vi "UserMgr-Window.vi"(8 "error in":errorcluster) -> (0 "error out":errorcluster)   [LabVIEW 2017, in "Login-UI.lvlib"]
uses:
  Login-UI.lvlib
  _Typedef/User-Info.ctl
  _Typedef/User-Role.ctl
  2fbc59fa-d6e3-46c3-98fb-aa3f40a50569.vi
  b49018c0-b0cc-4a1e-8c0a-6a6f7b5dc366.vi
  <userlib>/NEVSTOP-Programming-Palette/Configuration/ClusterCfgTable/Parse CfgTable(with DataName).vi
panel:
  in  "Exit":bool
  in  "Edit Button":bool
  in  "Add Button":bool
  in  "Delete Button":bool
  in  "Table":i32(listbox)
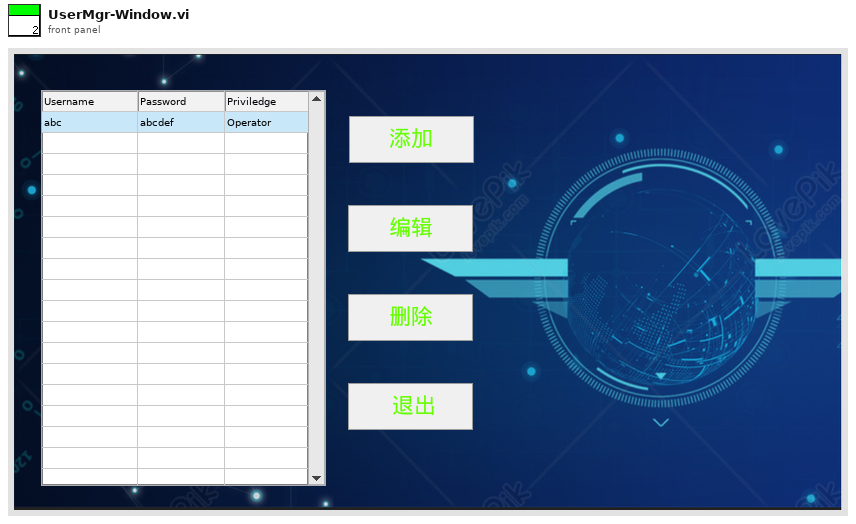
[diagram p1: front panel]
types:
  T1 = typedef "Login-UI.lvlib/User-Info.ctl" = cluster{"UserName":string, "Password":string, "Role":T2}
  T2 = typedef "Login-UI.lvlib/User-Role.ctl" = enum16{"INVALID", "Operator", "Engineer", "Admin"}
  T3 = enum32{"Invalid", "Standard", "Closed", "Hidden", "Minimized", "Maximized"}
  T4 = enum32{"invalid app kind", "Development System", "Run Time System", "Student Edition", "Embedded LabVIEW", "Evaluation", "Custom"}
  T5 = cluster{"Core":cluster{"Current VI Reference":refnum<vi>, "Close Panel on Exit?":bool}, "Your Boolean data":bool, "Your string data":string, "Table Ref":refnum<vi>}
  T6 = cluster{"Current VI Reference":refnum<vi>, "Close Panel on Exit?":bool}
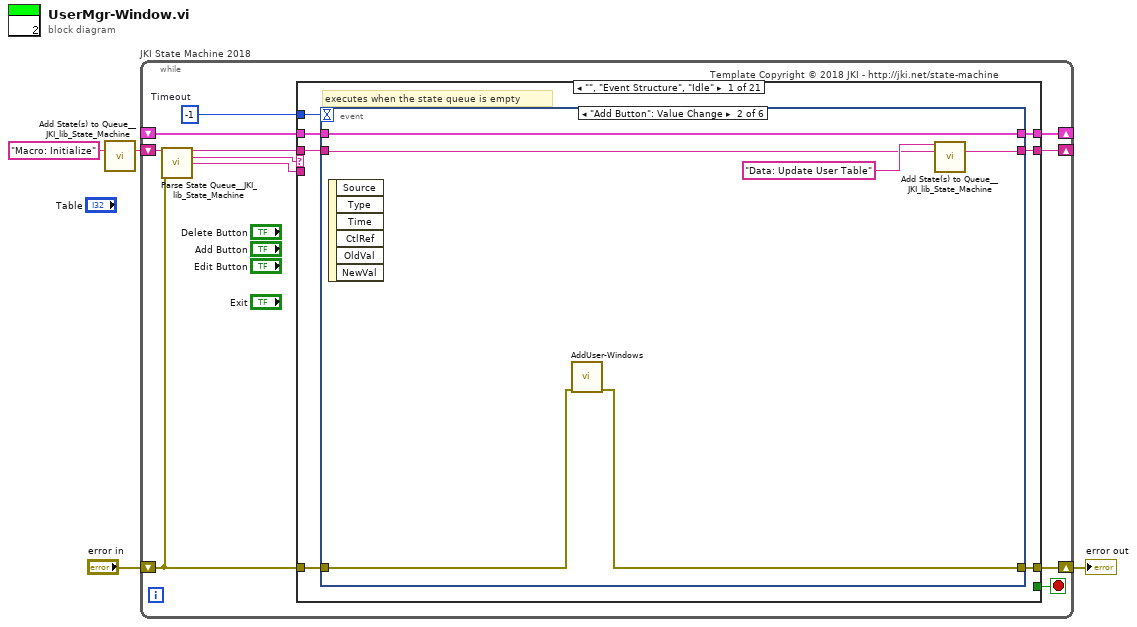
[diagram p0: block diagram]
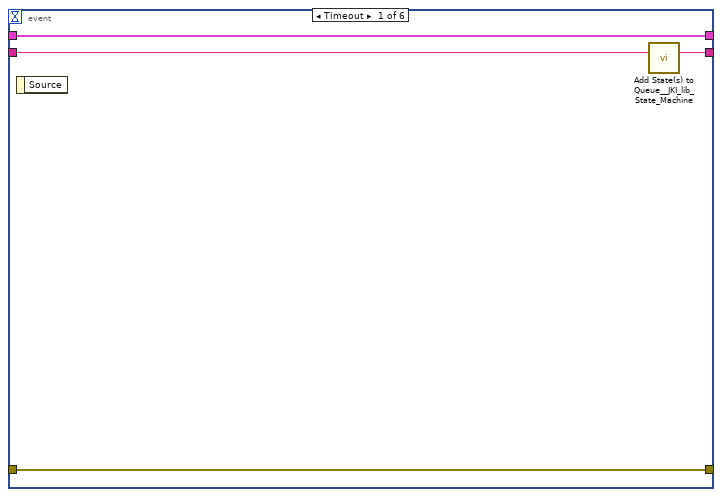
[diagram p2: hidden frame]
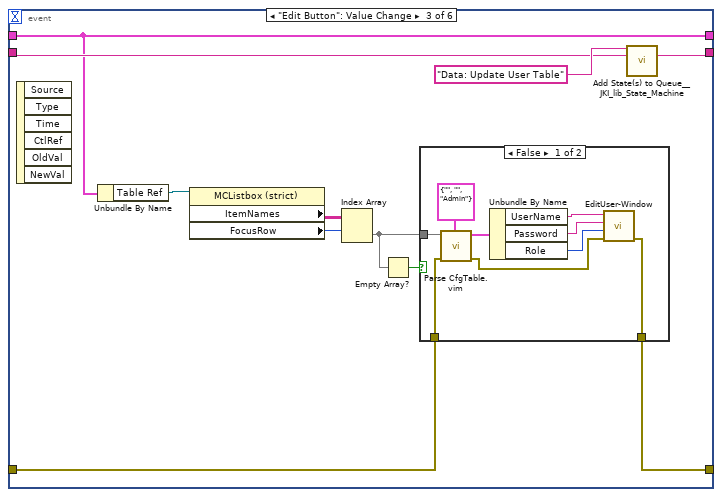
[diagram p3: hidden frame]
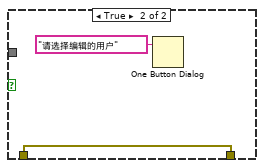
[diagram p4: hidden frame]
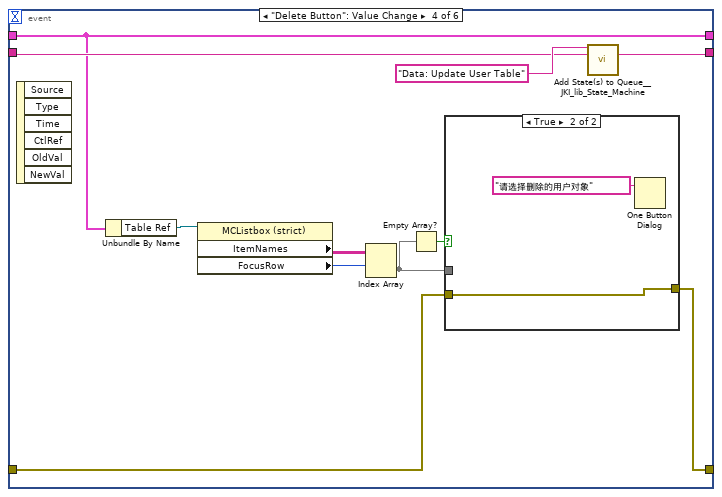
[diagram p5: hidden frame]
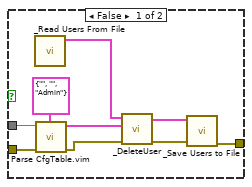
[diagram p6: hidden frame]
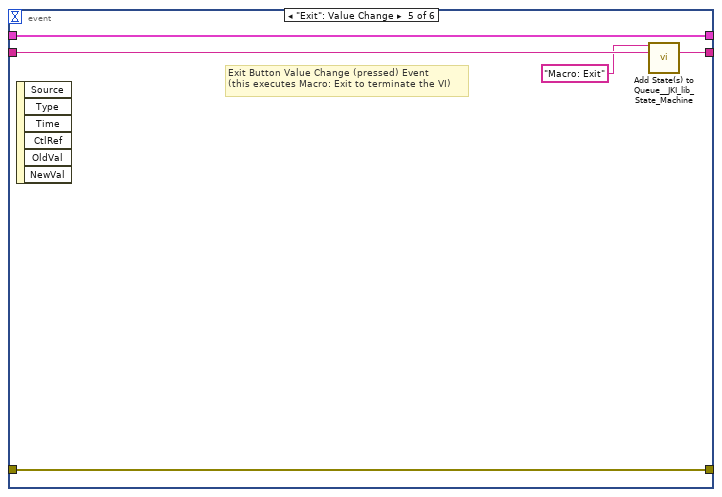
[diagram p7: hidden frame]
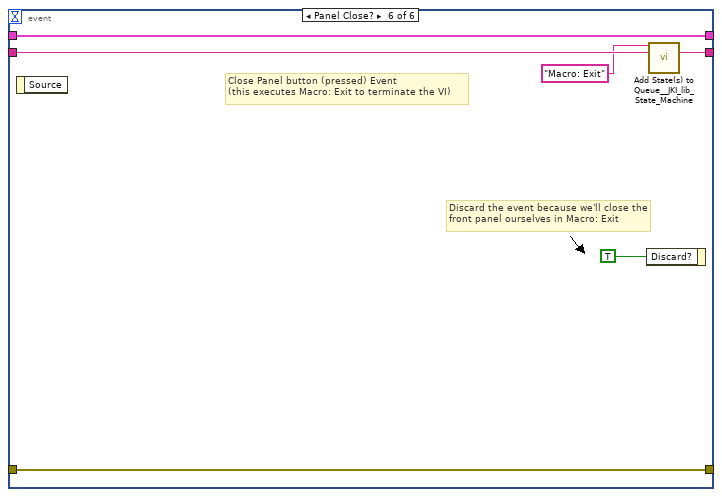
[diagram p8: hidden frame]
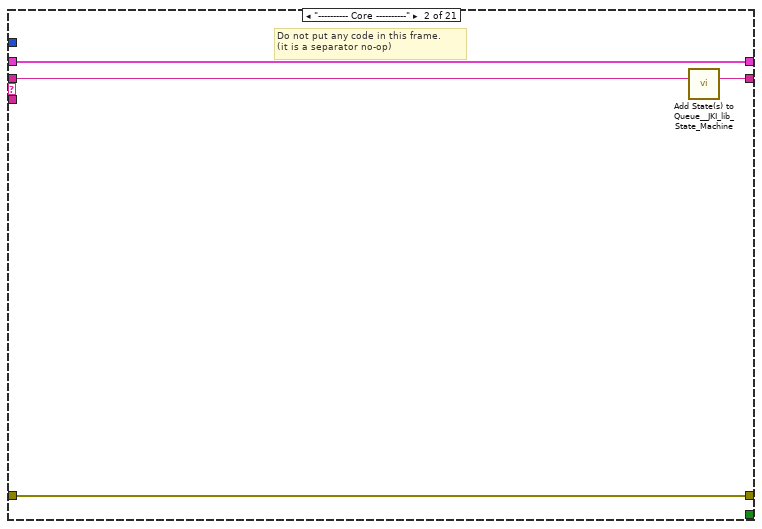
[diagram p9: hidden frame]
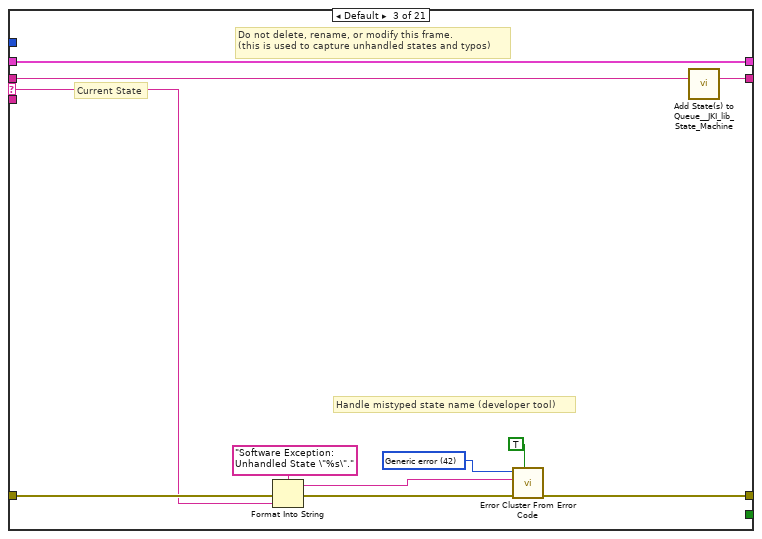
[diagram p10: hidden frame]
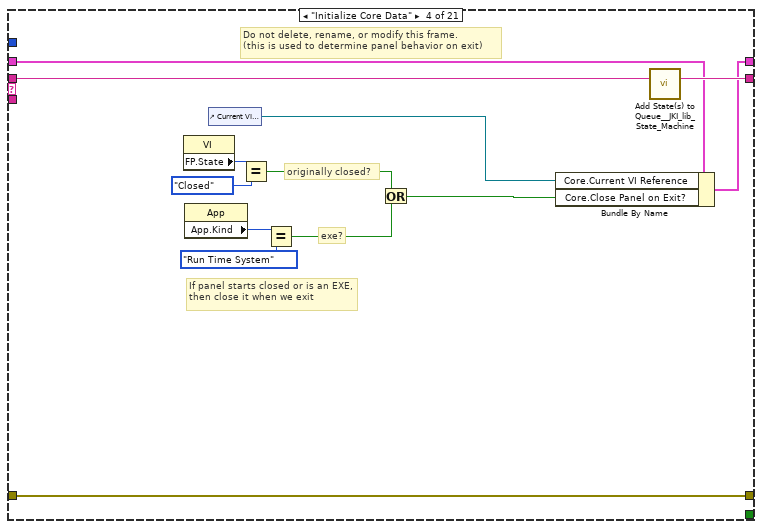
[diagram p11: hidden frame]
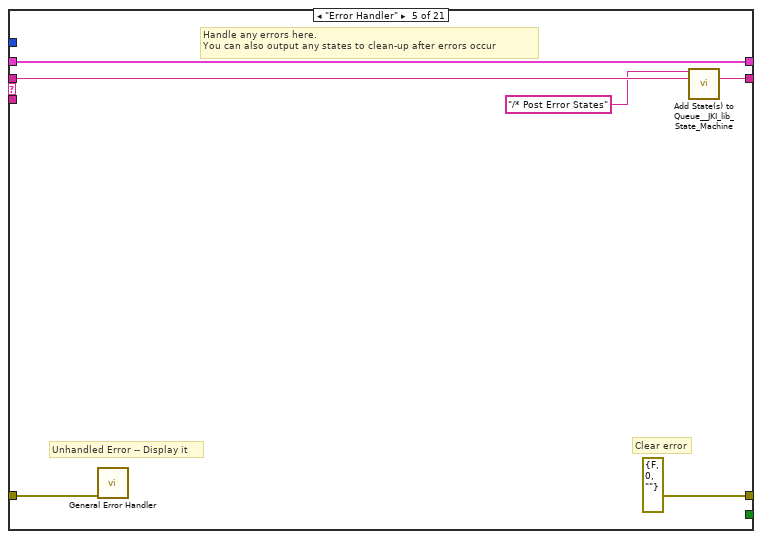
[diagram p12: hidden frame]
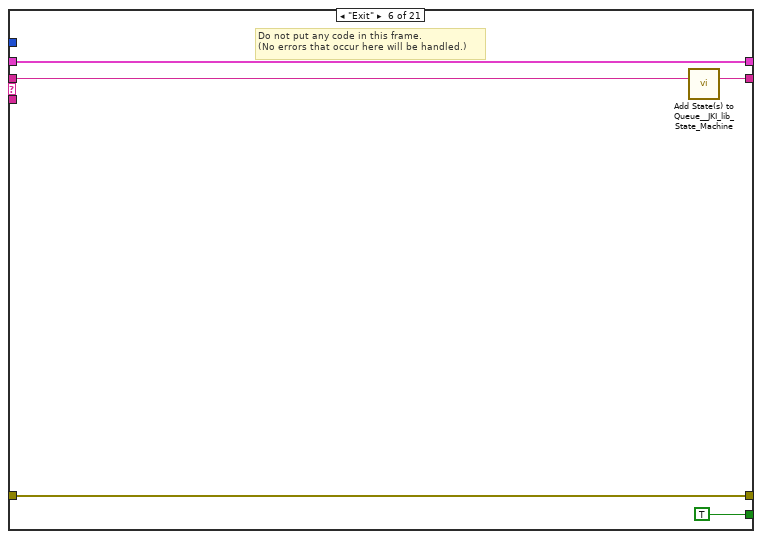
[diagram p13: hidden frame]
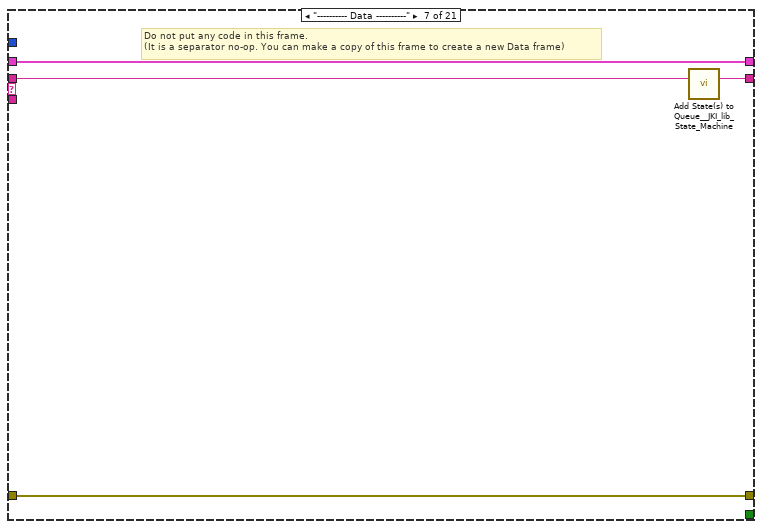
[diagram p14: hidden frame]
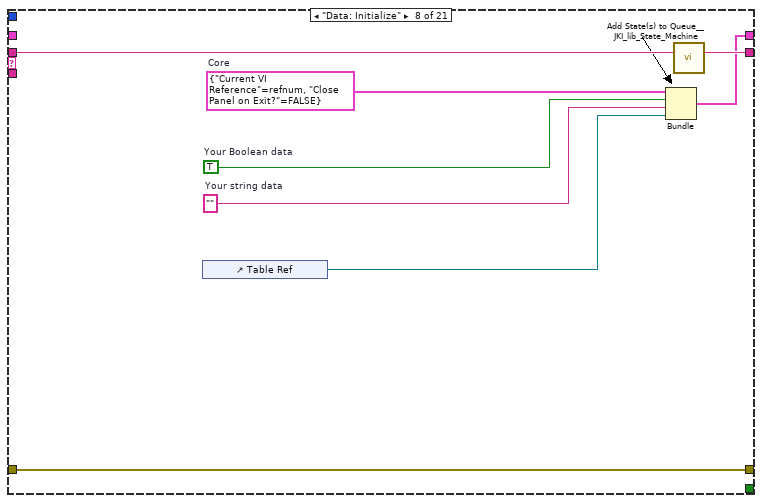
[diagram p15: hidden frame]
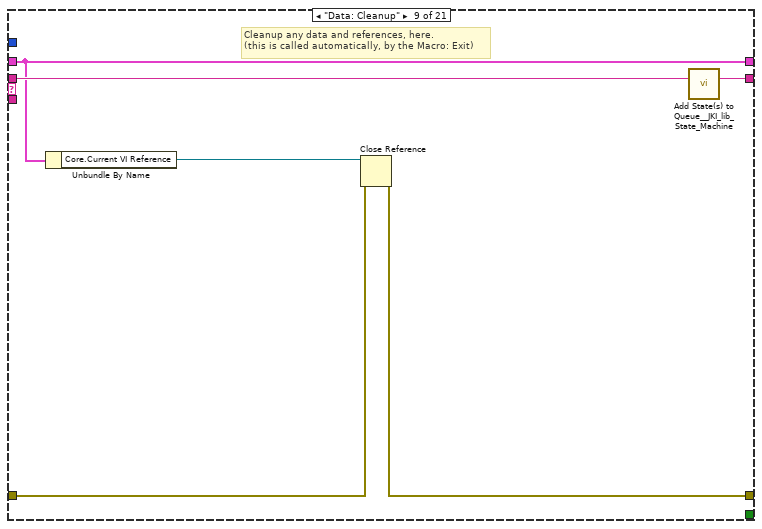
[diagram p16: hidden frame]
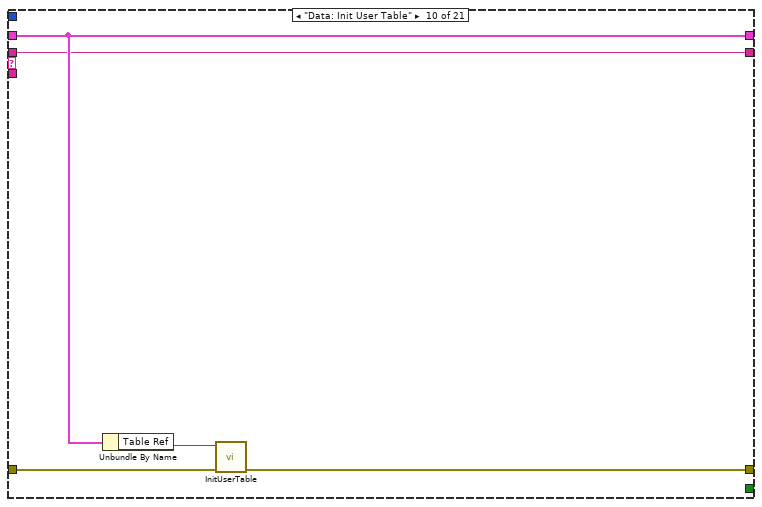
[diagram p17: hidden frame]
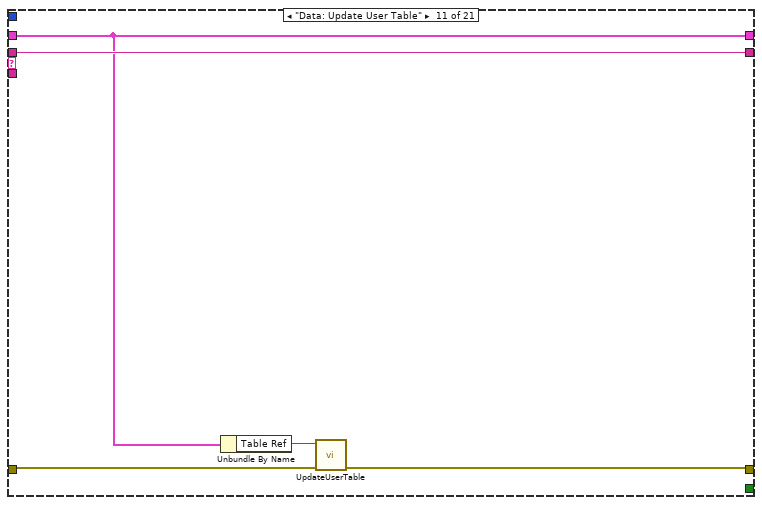
[diagram p18: hidden frame]
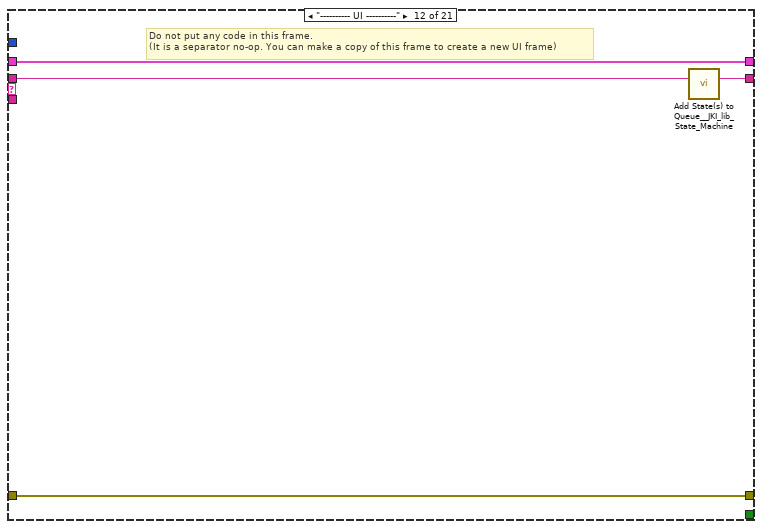
[diagram p19: hidden frame]
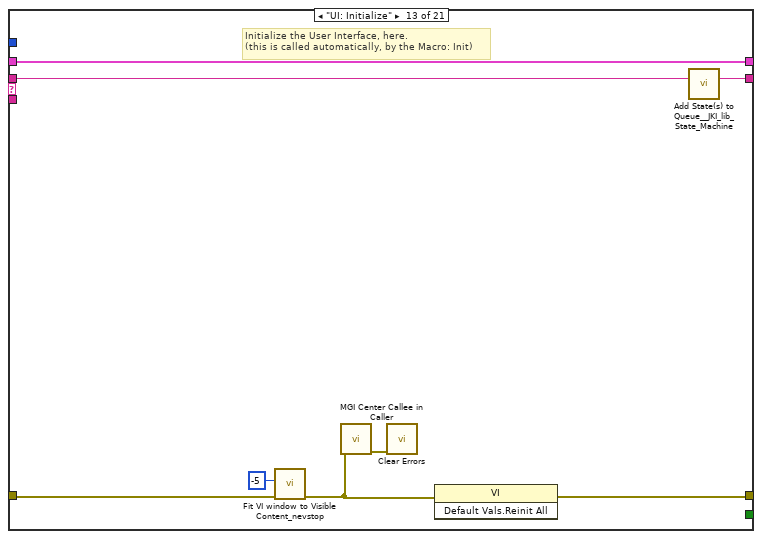
[diagram p20: hidden frame]
diagram:
  n1 = call <vilib>:"Add State(s) to Queue__JKI_lib_State_Machine.vi"("State(s) in (\"\")"="Macro: Initialize") -> ("States Out"=w4:string)  [unwired: 14 in]
  n2 = while "JKI State Machine 2018" {
    shift-right: [w8] -> _
    shift-left: _ -> [w7]
    shift-right: [w11] -> w1
    shift-left: "error in" -> [w5]
    shift-right: [w10] -> _
    shift-left: w4 -> [w12]
    stop <- w9 stop-if-true
    w6 = -1  # Timeout
    # "Template Copyright © 2018 JKI - http://jki.net/state-machine"
    n3 = call <vilib>:"Parse State Queue__JKI_lib_State_Machine.vi"("State Queue"=w12, "Error In (no error)"=w5) -> ("Remaining States"=w14:string, "Current State"=w15:string, "Arguments"=w13:string)  [unwired: 11 in]
    n4 = case shown="\"\", \"Event Structure\", \"Idle\"" w15 {
      selector: w15 -> [_ _ w92 _ _ _ _ _ _ _ _ _ _ _ _ _ _ _ _ _ _]
      tunnel: w14 -> [w22 w91 w96 w115 w121 w126 w130 w138 w144 w145 w151 w158 w166 w172 w183 w252 w257 w267 w271 w275 w279]
      tunnel: w13 -> [_ _ _ _ _ _ _ _ _ _ _ _ _ w167 w177 _ _ _ _ _ _]
      tunnel: w7 -> [w20 w88 w94 w108 w118 w124 w127 _ w139 w146 w150 w155 w164 w170 w179 w249 w254 w264 w268 w272 w276]
      tunnel: [w19 w89 w98 w112 errorcluster {"status"=FALSE, "code"=0, "source"=""} ("error out") w123 w128 w135 w140 w148 w153 w156 w161 w168 w180 w250 w255 w265 w269 w273 w277] -> w11
      tunnel: w5 -> [w18 w89 w97 w112 w117 w123 w128 w135 w141 w149 w154 w156 w162 w169 w181 w250 w255 w265 w269 w273 w277]
      tunnel: [w21 w90 w95 w114 w120 w125 w129 w137 w143 w145 w151 w157 w165 w171 w182 w251 w256 w266 w270 w274 w278] -> w10
      tunnel: [_ _ _ _ _ TRUE _ _ _ _ _ _ _ _ _ _ _ _ _ _ _] -> w9
      tunnel: [w17 w88 w94 w113 w118 w124 w127 w136 w139 w146 w150 w155 w164 w170 w179 w249 w254 w264 w268 w272 w276] -> w8
      tunnel: w6 -> [w16 _ _ _ _ _ _ _ _ _ _ _ _ _ _ _ _ _ _ _ _]
      frame "", "Event Structure", "Idle" {
        # "executes when the state queue is empty"
        n5 = event shown="[1] \"Add Button\": Value Change" {
          selector: _ -> [_ _ _ _ _ _]
          dyn-events: _ -> [_ _ _ _ _ _]
          timeout: w16 -> [_ _ _ _ _ _]
          tunnel: w22 -> [w26 w30 w41 w63 w81 w87]
          tunnel: [w25 w29 w42 w64 w80 w86] -> w21
          tunnel: w20 -> [w23 w32 w40 w59 w78 w84]
          tunnel: [w24 w27 w35 w55 w79 w85] -> w19
          tunnel: w18 -> [w24 w28 w36 w56 w79 w85]
          tunnel: [w23 w32 w40 w59 w78 w84] -> w17
          event Timeout {
            n6 = event-data() -> ()  [unwired: 1 in, 1 out]
            n7 = call <vilib>:"Add State(s) to Queue__JKI_lib_State_Machine.vi"("State(s) in (\"\")"=w26) -> ("States Out"=w25:string)  [unwired: 14 in]
          }
          event "Add Button": Value Change {
            n8 = event-data() -> ()  [unwired: 1 in, 6 out]
            n9 = call "AddUser-Windows.vi"("error in"=w28) -> ("error out"=w27:errorcluster)  [unwired: 10 in]
            n10 = call <vilib>:"Add State(s) to Queue__JKI_lib_State_Machine.vi"("State(s) in Front (\"\")"="Data: Update User Table", "State(s) in (\"\")"=w30) -> ("States Out"=w29:string)  [unwired: 13 in]
          }
          event "Edit Button": Value Change {
            n11 = event-data() -> ()  [unwired: 1 in, 6 out]
            n12 = Unbundle By Name(w40) -> ("Table Ref"=w39:refnum<vi>)
            n13 = property class="MCListbox (strict)"(reference=w39) -> ("ItemNames"=w38:string[][], "FocusRow"=w37:i32)  [unwired: 1 in, 2 out]
            n14 = Index Array(array=w38, index (row)=w37) -> (element=w33:string[])  [unwired: 1 in]
            n15 = Empty Array?(array=w33) -> (empty?=w34:bool)
            n16 = case shown="False" w34 {
              tunnel: w33 -> [w52 _]
              tunnel: w36 -> [w46 w53]
              tunnel: [w44 w53] -> w35
              frame False {
                n17 = call "Parse CfgTable.vim"("Cluster Configuration Typedef"=T1 {"UserName"="", "Password"="", "Role"=enum."Admin"} ("Cluster"), "error in (no error)"=w46, "CfgTable Row"=w52) -> ("error out"=w45:errorcluster, "Cluster Configuration Out"=w50:T1)  [unwired: 7 in]
                n18 = Unbundle By Name(w50) -> ("UserName"=w49:string, "Password"=w48:string, "Role"=w47:T2)
                n19 = call "EditUser-Window.vi"("error in"=w45, "权  限"=w47, "密  码"=w48, "用户名"=w49) -> ("error out"=w44:errorcluster)  [unwired: 7 in]
              }
              frame True {
                n20 = One Button Dialog(message="请选择编辑的用户") -> ()  [unwired: 1 in, 1 out]
              }
            }
            n21 = call <vilib>:"Add State(s) to Queue__JKI_lib_State_Machine.vi"("State(s) in Front (\"\")"="Data: Update User Table", "State(s) in (\"\")"=w41) -> ("States Out"=w42:string)  [unwired: 13 in]
          }
          event "Delete Button": Value Change {
            n22 = event-data() -> ()  [unwired: 1 in, 6 out]
            n23 = Unbundle By Name(w59) -> ("Table Ref"=w62:refnum<vi>)
            n24 = property class="MCListbox (strict)"(reference=w62) -> ("ItemNames"=w61:string[][], "FocusRow"=w60:i32)  [unwired: 1 in, 2 out]
            n25 = Index Array(array=w61, index (row)=w60) -> (element=w57:string[])  [unwired: 1 in]
            n26 = Empty Array?(array=w57) -> (empty?=w58:bool)
            n27 = case shown="True" w58 {
              tunnel: w57 -> [w74 _]
              tunnel: w56 -> [w67 w75]
              tunnel: [w66 w75] -> w55
              frame False {
                n28 = call "_Read Users From File.vi"() -> ("Array"=w72:T1[])  [unwired: 10 in, 1 out]
                n29 = call "Parse CfgTable.vim"("Cluster Configuration Typedef"=T1 {"UserName"="", "Password"="", "Role"=enum."Admin"} ("Cluster"), "error in (no error)"=w67, "CfgTable Row"=w74) -> ("error out"=w68:errorcluster, "Cluster Configuration Out"=w71:T1)  [unwired: 7 in]
                n30 = call "_DeleteUser.vi"("error in"=w68, "User"=w71, "User List"=w72) -> ("error out"=w69:errorcluster, "User List"=w70:T1[])  [unwired: 7 in]
                n31 = call "_Save Users to File.vi"("Error in"=w69, "Array"=w70) -> ("Error out"=w66:errorcluster)  [unwired: 9 in]
              }
              frame True {
                n32 = One Button Dialog(message="请选择删除的用户对象") -> ()  [unwired: 1 in, 1 out]
              }
            }
            n33 = call <vilib>:"Add State(s) to Queue__JKI_lib_State_Machine.vi"("State(s) in Front (\"\")"="Data: Update User Table", "State(s) in (\"\")"=w63) -> ("States Out"=w64:string)  [unwired: 13 in]
          }
          event "Exit": Value Change {
            # "Exit Button Value Change (pressed) Event\n(this executes Macro: Exit to terminate the VI)"
            n34 = event-data() -> ()  [unwired: 1 in, 6 out]
            n35 = call <vilib>:"Add State(s) to Queue__JKI_lib_State_Machine.vi"("State(s) in Front (\"\")"="Macro: Exit", "State(s) in (\"\")"=w81) -> ("States Out"=w80:string)  [unwired: 13 in]
          }
          event Panel Close? {
            # "Discard the event because we'll close the front panel ourselves in Macro: Exit"
            # "Close Panel button (pressed) Event\n(this executes Macro: Exit to terminate the VI)"
            n36 = event-data() -> ()  [unwired: 1 in, 1 out]
            n37 = event-data("Discard?"=TRUE) -> ()  [unwired: 1 in, 1 out]
            n38 = call <vilib>:"Add State(s) to Queue__JKI_lib_State_Machine.vi"("State(s) in Front (\"\")"="Macro: Exit", "State(s) in (\"\")"=w87) -> ("States Out"=w86:string)  [unwired: 13 in]
          }
        }
      }
      frame "---------- Core ----------" {
        # "Do not put any code in this frame.\n(it is a separator no-op)"
        n39 = call <vilib>:"Add State(s) to Queue__JKI_lib_State_Machine.vi"("State(s) in (\"\")"=w91) -> ("States Out"=w90:string)  [unwired: 14 in]
      }
      frame Default {
        w101 = 42 items=["No error", "Argument error", "Memory is full", "Out of zone", "End of file", "File already open", "Generic file I/O error", "File not found", "File permission error", "Disk is full", "Duplicate path", "Too many files open", "System feature not enabled", "Resource file not found", "Cannot add resource", "Resource not found", "Image not found", "Image memory error", "Pen does not exist", "Config type invalid", "Config token not found", "Config parse error", "Config memory error", "Bad external code format", "Bad external code offset", "External code not present", "Null window", "Destroy window error", "Null menu", "Print aborted", "Bad print record", "Print driver error", "Windows error during printing", "Memory error during printing", "Print dialog error", "Generic print error", "Invalid device refnum", "Device not found", "Device parameter error", "Device unit error", "Cannot open device", "Device call aborted", "Generic error", "Cancelled by user", "Object ID too low", "Object ID too high", "Object not in heap", "Unknown heap", "Unknown object (invalid DefProc)", "Unknown object (DefProc not in table)", "Message out of range", "Invalid (null) method", "Unknown message", "Manager call not supported", "Bad address", "Network operation in progress", "Network operation timed out", "Connection is busy", "Network attribute not supported", "Network error", "Address in use", "System out of memory", "Connection aborted", "Connection refused", "Not connected", "Already connected", "Connection closed", "Initialization error (interapplication manager)", "Bad occurrence", "Wait on unbound occurrence handler", "Occurrence queue overflow", "Datalog type conflict", "Unused", "Unrecognized type (interapplication manager)", "Memory corrupt", "Failed to make temporary DLL", "Old CIN version", "Drag socket not found", "Failed to load drop-object", "Failed to register OLE object", "Failed to release OLE object", "Format specifier type mismatch", "Unknown format specifier", "Too few format specifiers", "Too many format specifiers", "Scan failed", "Newer CIN version", "Error converting to variant", "Runtime menu error", "Password tampered", "Variant attribute not found", "Incompatible variant data type", "Event data is not available", "Event Store is not present", "Occurrence is not found", "Event Queue is not created", "Event info is not available", "Refnum passed is NULL", "Error retrieving Class GUID", "Error retrieving CoClass GUID", "Error retrieving TypeLib GUID.", "Bad built application magic bytes.", "Specific driver is different from the specific driver associated with the Logical Name.", "There is no session opened to the class driver.", "Max Error", "MAX - Error with config objects", "MAX - Error loading configuration", "MAX - Group not supported"]
        # "Current State"
        # "Do not delete, rename, or modify this frame.\n(this is used to capture unhandled states and typos)"
        # "Handle mistyped state name (developer tool)"
        n40 = Format Into String(format string="Software Exception: Unhandled State \"%s\"." ("message"), error in=w97, w92) -> (resulting string=w100:string, error out=w99:errorcluster)  [unwired: 1 in]
        n41 = call <vilib>:"Error Cluster From Error Code.vi"("show call chain? (False)"=TRUE, "error in (no error)"=w99, "error message (\"\")"=w100, "error code (0)"=w101) -> ("error out"=w98:errorcluster)  [unwired: 5 in]
        n42 = call <vilib>:"Add State(s) to Queue__JKI_lib_State_Machine.vi"("State(s) in (\"\")"=w96) -> ("States Out"=w95:string)  [unwired: 14 in]
      }
      frame "Initialize Core Data" {
        # "Do not delete, rename, or modify this frame.\n(this is used to determine panel behavior on exit)"
        # "originally closed?"
        # "exe?"
        # "If panel starts closed or is an EXE, then close it when we exit"
        n43 = property class="VI"() -> ("FP.State"=w105:T3)  [unwired: 2 in, 2 out]
        n44 = property class="App"() -> ("App.Kind"=w111:T4)  [unwired: 2 in, 2 out]
        n45 = control-ref of="Current VI Reference"() -> (w106:refnum<vi>)
        n46 = Equal?(x=w105, y=T3."Closed" ("Front Panel Window:State")) -> (x = y?=w103:bool)
        n47 = Equal?(x=w111, y=T4."Run Time System" ("Application:Kind")) -> (x = y?=w109:bool)
        n48 = Or(x=w103, y=w109) -> (x .or. y?=w107:bool)
        n49 = Bundle By Name(cluster=w108, "Core.Current VI Reference"=w106, "Core.Close Panel on Exit?"=w107) -> (w113:T5)
        n50 = call <vilib>:"Add State(s) to Queue__JKI_lib_State_Machine.vi"("State(s) in (\"\")"=w115) -> ("States Out"=w114:string)  [unwired: 14 in]
      }
      frame "Error Handler" {
        # "Unhandled Error -- Display it"
        # "Handle any errors here.\nYou can also output any states to clean-up after errors occur"
        # "Clear error"
        n51 = call <vilib>:"General Error Handler.vi"("error in (no error)"=w117) -> ()  [unwired: 10 in, 5 out]
        n52 = call <vilib>:"Add State(s) to Queue__JKI_lib_State_Machine.vi"("State(s) in Front (\"\")"="/* Post Error States", "State(s) in (\"\")"=w121) -> ("States Out"=w120:string)  [unwired: 13 in]
      }
      frame "Exit" {
        # "Do not put any code in this frame.\n(No errors that occur here will be handled.)"
        n53 = call <vilib>:"Add State(s) to Queue__JKI_lib_State_Machine.vi"("State(s) in (\"\")"=w126) -> ("States Out"=w125:string)  [unwired: 14 in]
      }
      frame "---------- Data ----------" {
        # "Do not put any code in this frame.\n(It is a separator no-op. You can make a copy of this frame to create a new Data frame)"
        n54 = call <vilib>:"Add State(s) to Queue__JKI_lib_State_Machine.vi"("State(s) in (\"\")"=w130) -> ("States Out"=w129:string)  [unwired: 14 in]
      }
      frame "Data: Initialize" {
        w132 = T6 {"Current VI Reference"=refnum, "Close Panel on Exit?"=FALSE}  # Core
        w134 = TRUE  # Your Boolean data
        w133 = ""  # Your string data
        n55 = control-ref of="Table Ref"() -> (w131:refnum<vi>)
        n56 = Bundle("Core"=w132, "Your Boolean data"=w134, "Your string data"=w133, "Table Ref"=w131) -> (w136:T5)  [unwired: 1 in]
        n57 = call <vilib>:"Add State(s) to Queue__JKI_lib_State_Machine.vi"("State(s) in (\"\")"=w138) -> ("States Out"=w137:string)  [unwired: 14 in]
      }
      frame "Data: Cleanup" {
        # "Cleanup any data and references, here.\n(this is called automatically, by the Macro: Exit)"
        n58 = Unbundle By Name(w139) -> ("Core.Current VI Reference"=w142:refnum<vi>)
        n59 = Close Reference(reference=w142, error in (no error)=w141) -> (error out=w140:errorcluster)
        n60 = call <vilib>:"Add State(s) to Queue__JKI_lib_State_Machine.vi"("State(s) in (\"\")"=w144) -> ("States Out"=w143:string)  [unwired: 14 in]
      }
      frame "Data: Init User Table" {
        n61 = Unbundle By Name(w146) -> ("Table Ref"=w147:refnum<vi>)
        n62 = call "InitUserTable.vi"("Error in"=w149, "User Table"=w147) -> ("error out"=w148:errorcluster)  [unwired: 9 in]
      }
      frame "Data: Update User Table" {
        n63 = Unbundle By Name(w150) -> ("Table Ref"=w152:refnum<vi>)
        n64 = call "UpdateUserTable.vi"("Error in"=w154, "User Table"=w152) -> ("error out"=w153:errorcluster)  [unwired: 9 in]
      }
      frame "---------- UI ----------" {
        # "Do not put any code in this frame.\n(It is a separator no-op. You can make a copy of this frame to create a new UI frame)"
        n65 = call <vilib>:"Add State(s) to Queue__JKI_lib_State_Machine.vi"("State(s) in (\"\")"=w158) -> ("States Out"=w157:string)  [unwired: 14 in]
      }
      frame "UI: Initialize" {
        # "Initialize the User Interface, here.\n(this is called automatically, by the Macro: Init)"
        n66 = call <userlib>:"Fit VI window to Visible Content_nevstop.vi"("error in (no error)"=w162, "border spacing (2 px)"=-5) -> ("error out"=w160:errorcluster)  [unwired: 4 in, 1 out]
        n67 = call <userlib>:"MGI Center Callee in Caller.vi"("Error In"=w160) -> ("Error Out"=w159:errorcluster)  [unwired: 10 in]
        n68 = call <vilib>:"Clear Errors.vi"("error in (no error)"=w159) -> ()  [unwired: 5 in, 2 out]
        n69 = invoke class="VI" method="Default Vals.Reinit All"(error in=w160) -> (error out=w161:errorcluster)  [unwired: 2 in, 2 out]
        n70 = call <vilib>:"Add State(s) to Queue__JKI_lib_State_Machine.vi"("State(s) in (\"\")"=w166) -> ("States Out"=w165:string)  [unwired: 14 in]
      }
      frame "UI: Cursor Set" {
        # "Argument"
        # "Set and Unset Cursor Busy.\n(Usage: \"UI: Cursor Set >> Busy|Idle\")"
        n71 = case shown="\"Idle\", Default" w167 {
          tunnel: w169 -> [w174 w176]
          tunnel: [w173 w175] -> w168
          frame "Idle", Default {
            n72 = call <vilib>:"Unset Busy.vi"("error in (no error)"=w174) -> ("error out"=w173:errorcluster)  [unwired: 10 in]
          }
          frame "Busy" {
            n73 = call <vilib>:"Set Busy.vi"("error in (no error)"=w176) -> ("error out"=w175:errorcluster)  [unwired: 9 in, 1 out]
          }
        }
        n74 = call <vilib>:"Add State(s) to Queue__JKI_lib_State_Machine.vi"("State(s) in (\"\")"=w172) -> ("States Out"=w171:string)  [unwired: 14 in]
      }
      frame "UI: Front Panel State" {
        # "Argument"
        # "Set Front Panel Open or Closed\n(Usage: \"UI: Front Panel State >> Open|Close\")"
        n75 = Unbundle By Name(w179) -> ("Core.Current VI Reference"=w178:refnum<vi>)
        n76 = case shown="\"Minimize\", \"Minimized\"" w177 {
          tunnel: w181 -> [w189 w204 w215 w228 w241]
          tunnel: [w191 w205 w217 w230 w243] -> w180
          tunnel: w178 -> [w190 w202 w216 w229 w242]
          frame "Open", "Standard", Default {
            w184 = T3."Standard" ("State")
            n77 = property class="VI"(reference=w190, error in=w189) -> (reference out=w187:refnum<vi>, error out=w188:errorcluster, "FP.State"=w186:T3)
            n78 = Not Equal?(x=w186, y=w184) -> (x != y?=w185:bool)
            n79 = case shown="True" w185 {
              tunnel: [w195 w197] -> w191
              tunnel: w188 -> [w194 w197]
              tunnel: w187 -> [w193 _]
              tunnel: w184 -> [w192 _]
              frame True {
                n80 = invoke class="VI" method="FP.Open"(reference=w193, error in=w194, "Activate"=TRUE, "State"=w192) -> (error out=w195:errorcluster)  [unwired: 1 in, 4 out]
              }
              frame False {
              }
            }
          }
          frame "Close", "Closed" {
            n81 = property class="VI"(reference=w202, error in=w204) -> (reference out=w201:refnum<vi>, error out=w203:errorcluster, "FP.State"=w199:T3)
            n82 = Not Equal?(x=w199, y=T3."Closed" ("Front Panel Window:State")) -> (x != y?=w198:bool)
            n83 = case shown="True" w198 {
              tunnel: [w206 w209] -> w205
              tunnel: w203 -> [w206 w208]
              tunnel: w201 -> [_ w207]
              frame False {
              }
              frame True {
                n84 = invoke class="VI" method="FP.Close"(reference=w207, error in=w208) -> (error out=w209:errorcluster)  [unwired: 1 in, 2 out]
              }
            }
          }
          frame "Hidden", "Hide" {
            w210 = T3."Hidden" ("State")
            n85 = property class="VI"(reference=w216, error in=w215) -> (reference out=w213:refnum<vi>, error out=w214:errorcluster, "FP.State"=w212:T3)
            n86 = Not Equal?(x=w212, y=w210) -> (x != y?=w211:bool)
            n87 = case shown="True" w211 {
              tunnel: [w221 w222] -> w217
              tunnel: w214 -> [w220 w222]
              tunnel: w213 -> [w219 _]
              tunnel: w210 -> [w218 _]
              frame True {
                n88 = invoke class="VI" method="FP.Open"(reference=w219, error in=w220, "State"=w218) -> (error out=w221:errorcluster)  [unwired: 2 in, 4 out]
              }
              frame False {
              }
            }
          }
          frame "Minimize", "Minimized" {
            w223 = T3."Minimized" ("State")
            n89 = property class="VI"(reference=w229, error in=w228) -> (reference out=w226:refnum<vi>, error out=w227:errorcluster, "FP.State"=w225:T3)
            n90 = Not Equal?(x=w225, y=w223) -> (x != y?=w224:bool)
            n91 = case shown="True" w224 {
              tunnel: [w234 w235] -> w230
              tunnel: w227 -> [w233 w235]
              tunnel: w226 -> [w232 _]
              tunnel: w223 -> [w231 _]
              frame True {
                n92 = invoke class="VI" method="FP.Open"(reference=w232, error in=w233, "State"=w231) -> (error out=w234:errorcluster)  [unwired: 2 in, 4 out]
              }
              frame False {
              }
            }
          }
          frame "Maximize", "Maximized" {
            w236 = T3."Maximized" ("State")
            n93 = property class="VI"(reference=w242, error in=w241) -> (reference out=w239:refnum<vi>, error out=w240:errorcluster, "FP.State"=w238:T3)
            n94 = Not Equal?(x=w238, y=w236) -> (x != y?=w237:bool)
            n95 = case shown="True" w237 {
              tunnel: [w247 w248] -> w243
              tunnel: w240 -> [w246 w248]
              tunnel: w239 -> [w245 _]
              tunnel: w236 -> [w244 _]
              frame True {
                n96 = invoke class="VI" method="FP.Open"(reference=w245, error in=w246, "State"=w244) -> (error out=w247:errorcluster)  [unwired: 2 in, 4 out]
              }
              frame False {
              }
            }
          }
        }
        n97 = call <vilib>:"Add State(s) to Queue__JKI_lib_State_Machine.vi"("State(s) in (\"\")"=w183) -> ("States Out"=w182:string)  [unwired: 14 in]
      }
      frame "---------- Macro ----------" {
        # "Do not put any code in this frame.\n(It is a separator no-op. You can make a copy of this frame to create a new Macro frame)"
        n98 = call <vilib>:"Add State(s) to Queue__JKI_lib_State_Machine.vi"("State(s) in (\"\")"=w252) -> ("States Out"=w251:string)  [unwired: 14 in]
      }
      frame "Macro: Initialize" {
        w253 = "Data: Initialize\nInitialize Core Data\nUI: Initialize\nUI: Front Panel State >> Open\nData: Init User Table\nData: Update User Table"  # Data: Initialize Initialize Core Data UI: Initialize UI: Front Panel State >> Open Data: Init User Table Data: Update User Table
        # "Initialization Macro\n(This is called once, when the VI starts)"
        n99 = call <vilib>:"Add State(s) to Queue__JKI_lib_State_Machine.vi"("State(s) in Front (\"\")"=w253, "State(s) in (\"\")"=w257) -> ("States Out"=w256:string)  [unwired: 13 in]
      }
      frame "Macro: Exit" {
        # "Exit Macro\n(This is called once, when the VI exits)"
        n100 = Unbundle By Name(w264) -> ("Core.Close Panel on Exit?"=w263:bool)
        n101 = Select(t="UI: Front Panel State >> Close", s=w263, f="") -> (s? t:f=w260:string)
        n102 = call <vilib>:"Add State(s) to Queue__JKI_lib_State_Machine.vi"("State(s) in (\"\")"=w260, "State(s) at Back (\"\")"="Data: Cleanup\nExit") -> ("States Out"=w258:string)  [unwired: 13 in]
        n103 = call <vilib>:"Add State(s) to Queue__JKI_lib_State_Machine.vi"("State(s) in Front (\"\")"=w258, "State(s) in (\"\")"=w267) -> ("States Out"=w266:string)  [unwired: 13 in]
      }
      frame "---------- New Category ----------" {
        # "Template Separator\n(You can make a copy of, or modify, this frame)"
        n104 = call <vilib>:"Add State(s) to Queue__JKI_lib_State_Machine.vi"("State(s) in (\"\")"=w271) -> ("States Out"=w270:string)  [unwired: 14 in]
      }
      frame "New Category: 1" {
        # "Your code here.\n(You can make a copy of, or modify, this frame)"
        n105 = call <vilib>:"Add State(s) to Queue__JKI_lib_State_Machine.vi"("State(s) in (\"\")"=w275) -> ("States Out"=w274:string)  [unwired: 14 in]
      }
      frame "New Category: 2" {
        # "Your code here.\n(You can make a copy of, or modify, this frame)"
        n106 = call <vilib>:"Add State(s) to Queue__JKI_lib_State_Machine.vi"("State(s) in (\"\")"=w279) -> ("States Out"=w278:string)  [unwired: 14 in]
      }
    }
  }
  "error out" <- w1
